vi "setup-camera-acquisition.vi"(9 "Image Size":T3={"H Bin"=1.0, "V Bin"=1.0, "Left"=1.0, "Right"=1024.0, "Top"=1.0, "Bottom"=1024.0} {"V Bin" min=0.0; "H Bin" min=0.0 step=1.0}, 10 "Laser Shutter":T6, 11 "Acquisition Parameters":T5={"Readout Mode"=enum."Image", "Set Acquisition Mode"=enum."Run till abort", "Trigger Mode"=enum."Internal", "Exposure Time (sec)"=0.3, "Accumulation Cycle (s)"=1.0, "Kinetic Cycle Time (s)"=0.0, "Number of Kinetics"=1, "Number of Accumulations"=1, "Set VS Speed"=6.5, "Pixel Rate"=enum."EM CCD 1 Mhz 16 bits", "V Shift Amplitude"=enum."normal", "Preamp Gain"=enum."2.4", "Single Track Settings"={"centre"=0, "height"=1}, "EM CCD Gain"=300, "High Capacity?"=FALSE} {"EM CCD Gain" scale=0.01..300.0; "Single Track Settings"."centre" min=0 max=1024; "Single Track Settings"."height" min=1 max=1024; "Exposure Time (sec)" scale=0.001..10.0 scale format="%#_1g"; "Set VS Speed" min=0.0 format="%#_2f"}) -> (0 "Error Out":errorcluster, 1 "Continue with \nacquisition?":bool, 2 "Image Size Out":T2, 3 "File properties":T4)   [LabVIEW 2014]
uses:
  Shutter Control/Shutter SubVIs/ctts/laser shutters.ctl
  SubVIs/ctt's/Camera Setup Acquisition.ctl
  SubVIs/ctt's/Image size and binning.ctl
  Shutter Control/Shutter SubVIs/ctts/user event shutter global.ctl
  SubVIs/ctt's/image-acquision 2.ctl
  SubVIs/Globals/Initilize Globals.vi
panel:
  out "Pixels Out":i32[](array[numeric])
  in  "Preview Type":T1(radio)
  out "Y Pixel Size":u16
  out "X Pixel Size":u16
  in  "Adjust Image Size":bool
  in  "Set to AOI":bool
  in  "Set to 512 x 300":bool
  in  "Set to Maximum":bool
  in  "Number of preview \nwindows":i32=1 min=0 max=10
  in  "End Program?":bool
  in  "Camera \nShutter":bool
  out "Image":T7(plugin-control)
  # "Exit Parameters"
  # "****Configure Prior to Running Program****"
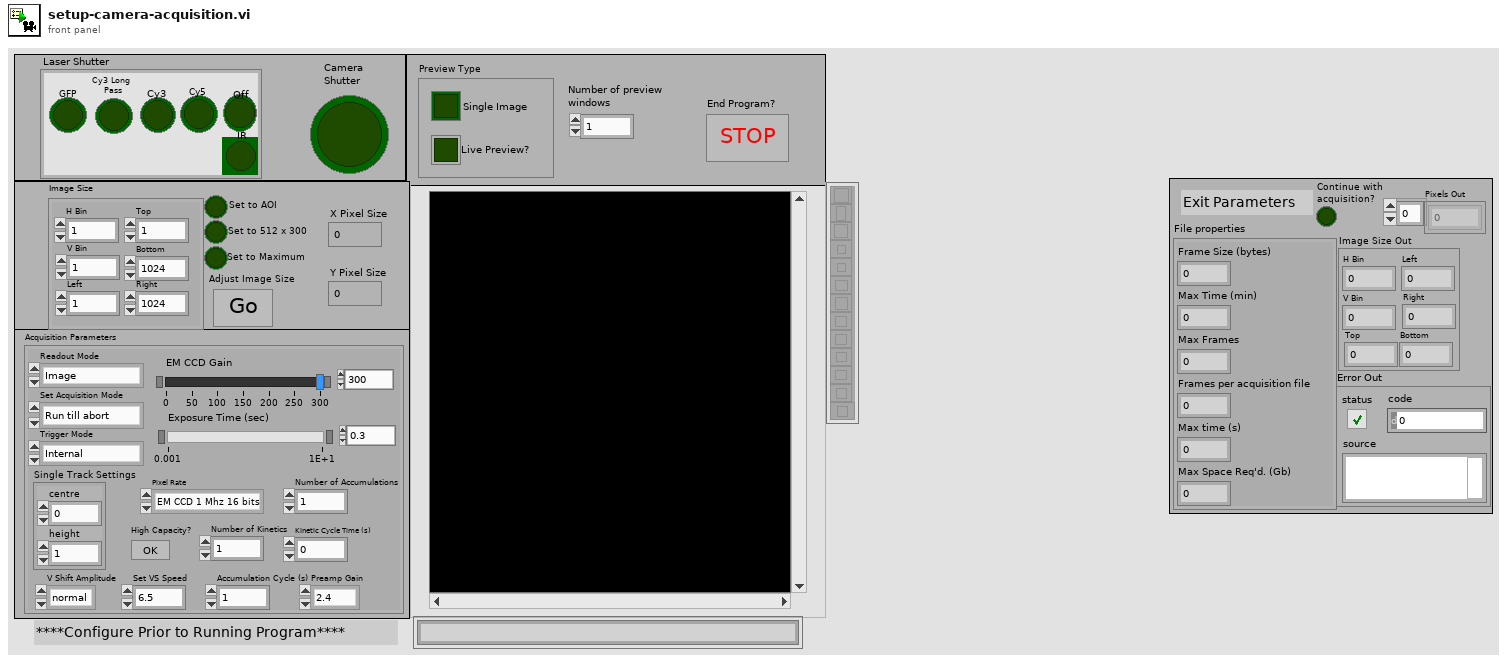
[diagram p1: front panel]
types:
  T1 = enum32{"No Selection", "Live Preview?", "Single Image"}
  T2 = cluster{"H Bin":dbl, "V Bin":dbl, "Left":dbl, "Right":dbl, "Top":dbl, "Bottom":dbl}
  T3 = typedef "Image size and binning.ctl" = cluster{"H Bin":dbl, "V Bin":dbl, "Left":dbl, "Right":dbl, "Top":dbl, "Bottom":dbl}
  T4 = cluster{"Frame Size (bytes)":i32, "Max Time (min)":i32, "Max Frames":i32, "Frames per acquisition file":i32, "Max time (s)":i32, "Max Space Req'd. (Gb)":dbl}
  T5 = typedef "Camera Setup Acquisition.ctl" = cluster{"Readout Mode":enum16{"Full Vertical Binning", "Multi-Track", "Random-Track", "Single-Track", "Image"}, "Set Acquisition Mode":enum16{"(do nothing)", "Single Scan", "Accumulate", "Kinetics", "Fast Kinetics", "Run till abort"}, "Trigger Mode":enum16{"Internal", "External"}, "Exposure Time (sec)":sgl, "Accumulation Cycle (s)":dbl, "Kinetic Cycle Time (s)":dbl, "Number of Kinetics":i32, "Number of Accumulations":i32, "Set VS Speed":dbl, "Pixel Rate":enum16{"EM CCD 10 Mhz 14 bits", "EM CCD 5 Mhz 14 bits", "EM CCD 3 Mhz 14 bits", "EM CCD 1 Mhz 16 bits", "Standard CCD 3 Mhz 14 bits", "Standard CCD 1 Mhz 16 bits"}, "V Shift Amplitude":enum16{"normal", "+1", "+2", "+3", "+4"}, "Preamp Gain":enum16{"1.0", "2.4", "5.0"}, "Single Track Settings":cluster{"centre":i32, "height":i32}, "EM CCD Gain":u16, "High Capacity?":bool}
  T6 = typedef "laser shutters.ctl" = enum32{"No Selection", "GFP", "Cy3 Long \nPass", "Cy3", "Cy5", "Off", "IR"}
  T7 = typedef "IMAQ Image.ctl" = refnum<image>
  T8 = enum32{"Invalid", "Standard", "Closed", "Hidden", "Minimized", "Maximized"}
  T9 = typedef "user event shutter global.ctl" = cluster{"Camera Shutter":bool, "Laser Shutter":enum32{"No Selection", "GFP", "Cy3 Long \nPass", "Cy3", "Cy5", "Off", "IR"}}
  T10 = enum32{"No Selection", "GFP", "Cy3 Long \nPass", "Cy3", "Cy5", "Off", "IR"}
  T11 = typedef "image-acquision 2.ctl" = u32
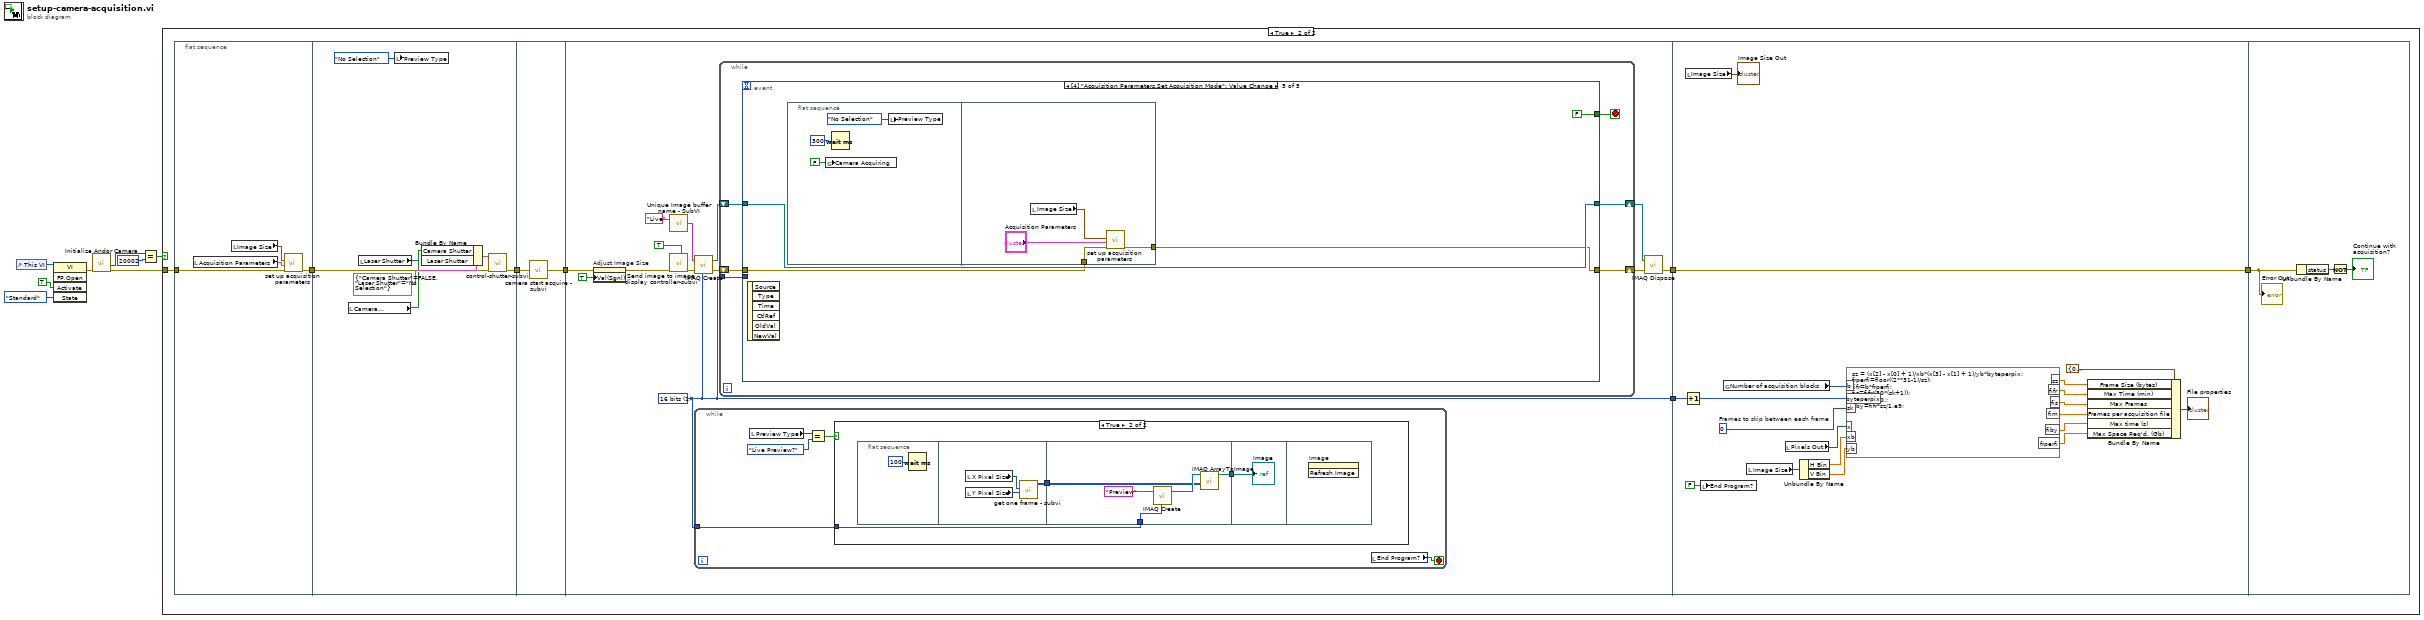
[diagram p0: block diagram]
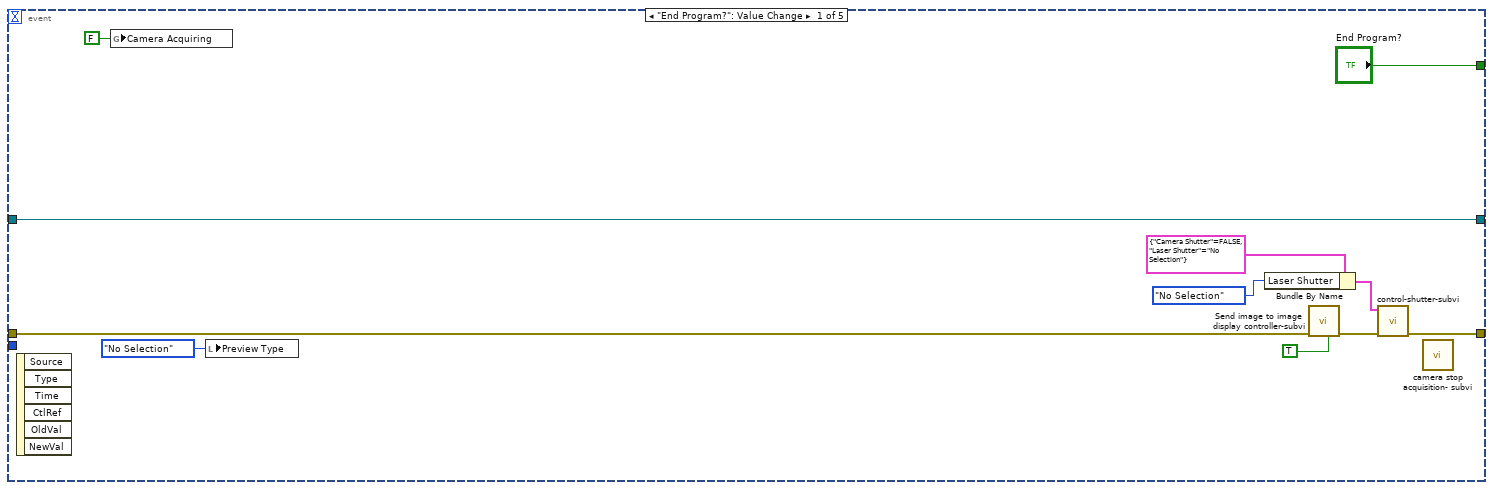
[diagram p4: hidden frame]
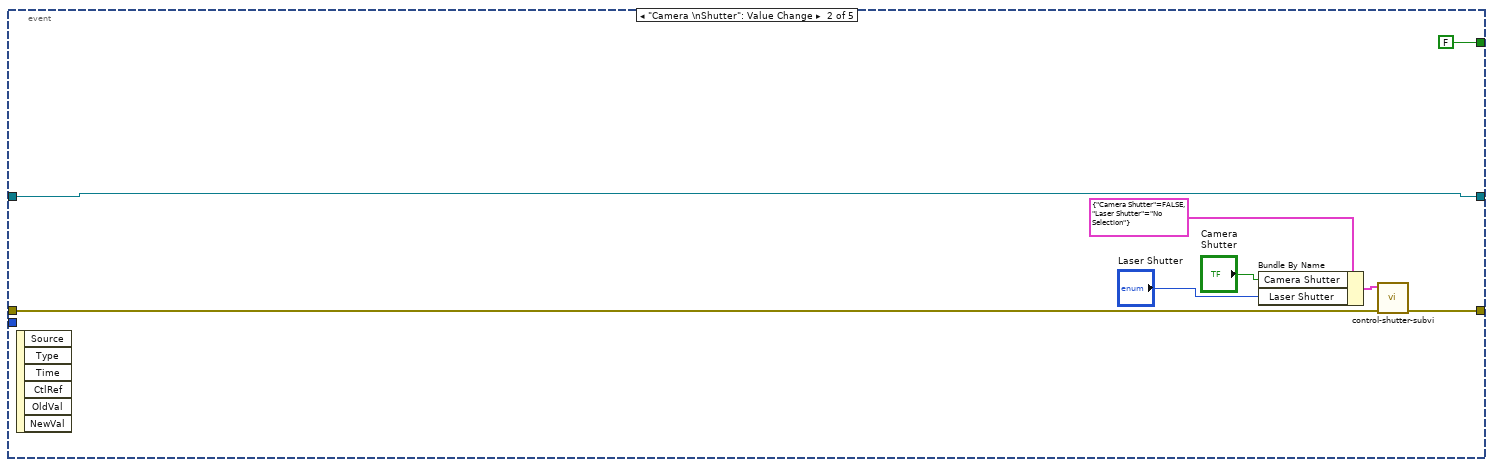
[diagram p5: hidden frame]
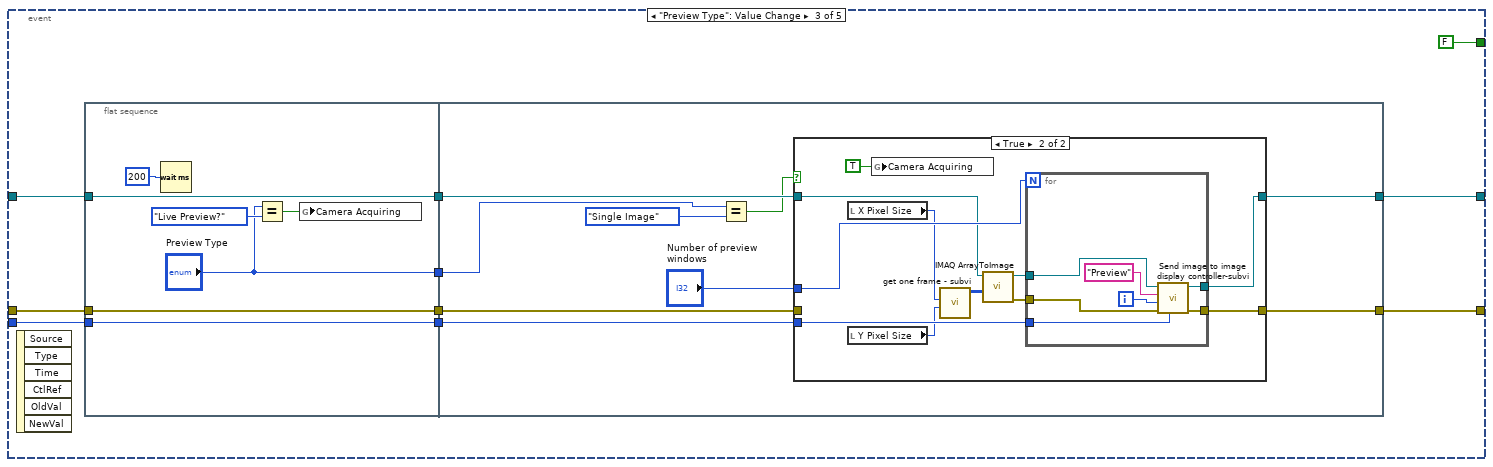
[diagram p6: hidden frame]
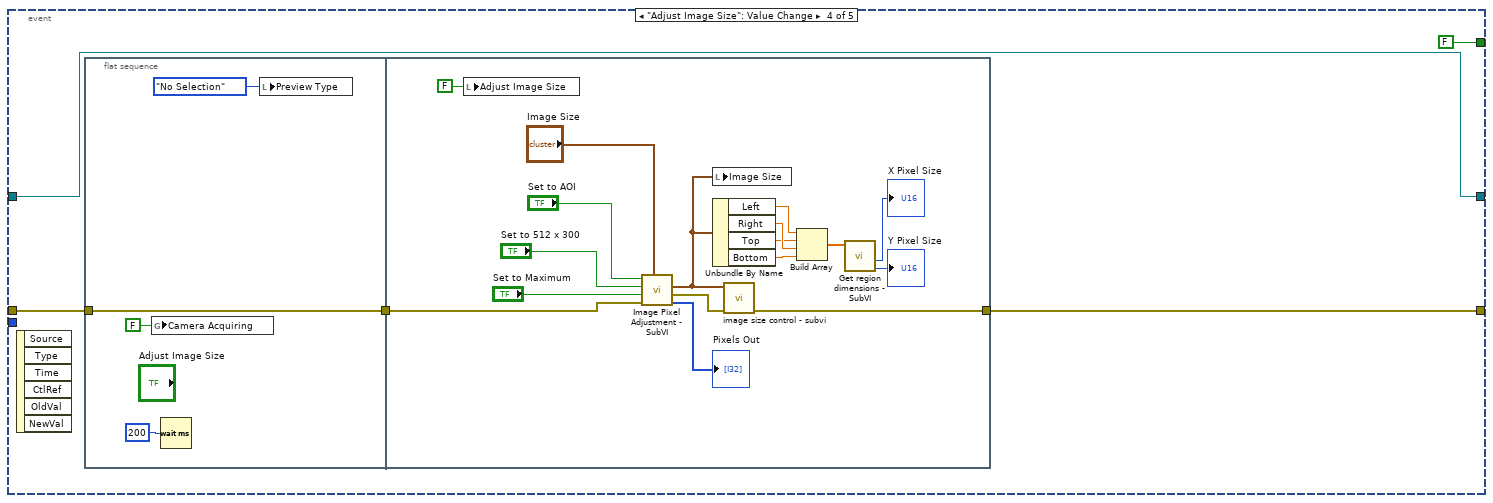
[diagram p8: hidden frame]
diagram:
  n1 = control-ref of="This VI"() -> (w8:refnum<vi>)
  n2 = invoke class="VI" method="FP.Open"(reference=w8, "Activate"=TRUE ("Activate?"), "State"=T8."Standard") -> (error out=w5:errorcluster)  [unwired: 2 in, 4 out]
  n3 = call "Initialize Andor Camera.vi"("error in (no error)"=w5) -> ("Error Out 2"=w1:errorcluster, "Drv Success?"=w4:i32)  [unwired: 9 in]
  n4 = Equal?(x=w4, y=20002) -> (x = y?=w2:bool)
  n5 = case shown="True" w2 {
    tunnel: w1 -> [_ w9]
    frame False {
    }
    frame True {
      n6 = flat-sequence {
        tunnel: [w18] -> w15
        tunnel: w9 -> [w17]
        tunnel: [w22] -> w14
        tunnel: w15 -> [w21]
        tunnel: w14 -> [w28]
        tunnel: [w27] -> w13
        tunnel: [w29] -> w12
        tunnel: w13 -> [w38]
        tunnel: [w40] -> w11
        tunnel: w12 -> [w184]
        tunnel: [w170] -> w10
        tunnel: w11 -> [w170]
        tunnel: w10 -> [w187]
        frame #0 {
          n7 = local read "Acquisition Parameters"() -> (w16:T5)
          n8 = local read "Image Size"() -> (w19:T3)
          n9 = call "set up acquisition parameters.vi"("error in (no error)"=w17, "Acquisition Parameters"=w16, "Image Size"=w19) -> ("error out"=w18:errorcluster)  [unwired: 3 in, 3 out]
        }
        frame #1 {
          n10 = local read "Camera \nShutter"() -> (w24:bool)
          n11 = local read "Laser Shutter"() -> (w23:T6)
          n12 = local write "Preview Type"(T1."No Selection" ("Preview Type")) -> ()
          n13 = Bundle By Name(cluster=T9 {"Camera Shutter"=FALSE, "Laser Shutter"=enum."No Selection"} ("Shutter Control"), "Camera Shutter"=w24, "Laser Shutter"=w23) -> (w25:T9)
          n14 = call "control-shutter-subvi.vi"("Error In"=w21, "Shutter Control"=w25) -> ("Error Out"=w22:errorcluster)  [unwired: 9 in]
        }
        frame #2 {
          n15 = call "camera start acquire - subvi.vi"("error in"=w28) -> ("error out"=w27:errorcluster)
        }
        frame #3 {
          w29 = T11 1 items=["8 bits", "16 bits", "Float", "Complex", "RGB", "HSL"] ("Image Type")
          n16 = property on="Adjust Image Size" class="Bool (strict)"(error in=w38, "Val(Sgnl)"=TRUE ("Value (Signaling)")) -> (error out=w32:errorcluster)  [unwired: 1 in, 1 out]
          n17 = call "Unique Image buffer name - SubVI.vi"("Buffer  base name"="Live") -> ("Image Name"=w35:string)  [unwired: 1 in]
          n18 = call "Send image to image display controller-subvi.vi"("error in"=w32, "Start display controller?"=TRUE) -> ("error out"=w31:errorcluster)  [unwired: 7 in, 1 out]
          n19 = call "IMAQ Create"("Image Name"=w35, "Image Type"=w29, "error in (no error)"=w31) -> ("New Image"=w33:T7, "error out"=w34:errorcluster)  [unwired: 1 in, 1 out]
          n20 = while {
            tunnel: w29 -> [w42]
            stop <- w46 stop-if-true
            n21 = local read "Preview Type"() -> (w45:T1)
            n22 = Equal?(x=w45, y=T1."Live Preview?" ("Preview Type")) -> (x = y?=w44:bool)
            n23 = case shown="True" w44 {
              tunnel: w42 -> [_ w47]
              frame False {
              }
              frame True {
                n24 = flat-sequence {
                  tunnel: [w51] -> w48
                  tunnel: [w56] -> w49
                  tunnel: w48 -> [w55]
                  tunnel: w47 -> [w54]
                  tunnel: w49 -> [w59]
                  frame #0 {
                    n25 = Wait (ms)(milliseconds to wait=u32 100) -> ()  [unwired: 1 out]
                  }
                  frame #1 {
                    n26 = local read "X Pixel Size"() -> (w52:u16)
                    n27 = local read "Y Pixel Size"() -> (w53:u16)
                    n28 = call "get one frame - subvi.vi"("Image Height"=w53, "Image Width"=w52) -> ("Image Array"=w51:i32[][])  [unwired: 9 in]
                  }
                  frame #2 {
                    n29 = call "IMAQ Create"("Image Name"="Preview", "Image Type"=w54) -> ("New Image"=w57:T7)  [unwired: 3 in, 1 out]
                    n30 = call "IMAQ ArrayToImage"("Image Pixels (I16)"=w55, "Image"=w57) -> ("Image Out"=w56:T7)  [unwired: 8 in, 1 out]
                  }
                  frame #3 {
                    "Image" <- w59
                  }
                  frame #4 {
                    n31 = invoke on="Image" class="ImageControl" method="Refresh Image"() -> ()  [unwired: 3 in, 3 out]
                  }
                }
              }
            }
            n32 = local read "End Program?"() -> (w46:bool)
          }
          n33 = while {
            tunnel: w29 -> [w64]
            shift-right: [w61] -> w41
            shift-left: w34 -> [w62]
            shift-right: [w60] -> w37
            shift-left: w33 -> [w63]
            stop <- w65 stop-if-true
            n34 = event shown="[4] \"Acquisition Parameters.Set Acquisition Mode\": Value Change" {
              selector: _ -> [_ _ _ _ _]
              dyn-events: _ -> [_ _ _ _ _]
              timeout: _ -> [_ _ _ _ _]
              tunnel: ["End Program?" FALSE ("Stop Preview?") FALSE ("Stop Preview?") FALSE ("Stop Preview?") FALSE ("Stop Preview?")] -> w65
              tunnel: w64 -> [_ _ w94 _ _]
              tunnel: w63 -> [w75 w77 w93 w134 w160]
              tunnel: [w75 w77 w91 w134 w160] -> w60
              tunnel: w62 -> [w74 w79 w89 w133 w158]
              tunnel: [w66 w78 w90 w132 w157] -> w61
              event "End Program?": Value Change {
                n35 = event-data() -> ()  [unwired: 1 in, 6 out]
                n36 = global write "Initilize Globals.vi" "Camera Acquiring"(FALSE) -> ()
                n37 = local write "Preview Type"(T1."No Selection" ("Preview Type")) -> ()
                n38 = Bundle By Name(cluster=T9 {"Camera Shutter"=FALSE, "Laser Shutter"=enum."No Selection"} ("Shutter Control"), "Laser Shutter"=T10."No Selection") -> (w68:T9)
                n39 = call "Send image to image display controller-subvi.vi"("error in"=w74, "Quit display controller?"=TRUE) -> ("error out"=w67:errorcluster)  [unwired: 7 in, 1 out]
                n40 = call "control-shutter-subvi.vi"("Error In"=w67, "Shutter Control"=w68) -> ("Error Out"=w66:errorcluster)  [unwired: 9 in]
                n41 = call "camera stop acquisition- subvi.vi"() -> ()  [unwired: 1 in]
              }
              event "Camera \nShutter": Value Change {
                n42 = event-data() -> ()  [unwired: 1 in, 6 out]
                n43 = Bundle By Name(cluster=T9 {"Camera Shutter"=FALSE, "Laser Shutter"=enum."No Selection"} ("Shutter Control"), "Camera Shutter"="Camera \nShutter", "Laser Shutter"="Laser Shutter") -> (w81:T9)
                n44 = call "control-shutter-subvi.vi"("Error In"=w79, "Shutter Control"=w81) -> ("Error Out"=w78:errorcluster)  [unwired: 9 in]
              }
              event "Preview Type": Value Change {
                n45 = event-data() -> ()  [unwired: 1 in, 6 out]
                n46 = flat-sequence {
                  tunnel: w89 -> [w99]
                  tunnel: w93 -> [w100]
                  tunnel: w94 -> [w101]
                  tunnel: [w101] -> w88
                  tunnel: [w100] -> w87
                  tunnel: [w99] -> w86
                  tunnel: ["Preview Type"] -> w85
                  tunnel: [w107] -> w91
                  tunnel: [w106] -> w90
                  tunnel: w88 -> [w110]
                  tunnel: w87 -> [w109]
                  tunnel: w86 -> [w105]
                  tunnel: w85 -> [w102]
                  frame #0 {
                    n47 = Wait (ms)(milliseconds to wait=u32 200) -> ()  [unwired: 1 out]
                    n48 = Equal?(x="Preview Type", y=T1."Live Preview?" ("Preview Type")) -> (x = y?=w95:bool)
                    n49 = global write "Initilize Globals.vi" "Camera Acquiring"(w95) -> ()
                  }
                  frame #1 {
                    n50 = Equal?(x=w102, y=T1."Single Image" ("Preview Type")) -> (x = y?=w104:bool)
                    n51 = case shown="True" w104 {
                      tunnel: w110 -> [_ w122]
                      tunnel: w109 -> [w112 w119]
                      tunnel: "Number of preview \nwindows" -> [_ w123]
                      tunnel: [w112 w120] -> w107
                      tunnel: [w111 w121] -> w106
                      tunnel: w105 -> [w111 _]
                      frame False {
                      }
                      frame True {
                        n52 = local read "X Pixel Size"() -> (w115:u16)
                        n53 = local read "Y Pixel Size"() -> (w114:u16)
                        n54 = global write "Initilize Globals.vi" "Camera Acquiring"(TRUE ("Camera Acquiring")) -> ()
                        n55 = call "get one frame - subvi.vi"("Image Height"=w114, "Image Width"=w115) -> ("Image Array"=w116:i32[][])  [unwired: 9 in]
                        n56 = call "IMAQ ArrayToImage"("Image Pixels (I16)"=w116, "Image"=w119) -> ("error out"=w117:errorcluster, "Image Out"=w118:T7)  [unwired: 4 in, 4 out]
                        n57 = for {
                          N: w123 -> [_]
                          tunnel: [w130] -> w121
                          tunnel: w117 -> [w129]
                          tunnel: w118 -> [w128]
                          tunnel: w122 -> [w126]
                          tunnel: [w125] -> w120
                          i -> [w127]
                          n58 = call "Send image to image display controller-subvi.vi"("Image"=w128, "Window Title"="Preview", "Window Number"=w127, "error in"=w129, "Image Type"=w126) -> ("Image Out"=w125:T7, "error out"=w130:errorcluster)  [unwired: 4 in]
                        }
                      }
                    }
                  }
                }
              }
              event "Adjust Image Size": Value Change {
                n59 = event-data() -> ()  [unwired: 1 in, 6 out]
                n60 = flat-sequence {
                  tunnel: w133 -> [w139]
                  tunnel: [w139] -> w131
                  tunnel: [w155] -> w132
                  tunnel: w131 -> [w156]
                  frame #0 {
                    n61 = global write "Initilize Globals.vi" "Camera Acquiring"(FALSE) -> ()
                    n62 = Wait (ms)(milliseconds to wait=u32 200) -> ()  [unwired: 1 out]
                    n63 = local write "Preview Type"(T1."No Selection" ("Preview Type")) -> ()
                  }
                  frame #1 {
                    n64 = local write "Adjust Image Size"(FALSE ("Adjust Image Size")) -> ()
                    n65 = call "Image Pixel Adjustment - SubVI.vi"("Image Size"="Image Size", "error in"=w156, "Set to Maximum"="Set to Maximum", "Set to 512 x 300"="Set to 512 x 300", "Set to AOI"="Set to AOI") -> ("Pixels Out"=→"Pixels Out":i32[], "Error Out (no error)"=w149:errorcluster, "Image Size 2"=w148:T2)  [unwired: 4 in]
                    n66 = local write "Image Size"(w148) -> ()
                    n67 = Unbundle By Name(w148) -> ("Left"=w146:dbl, "Right"=w141:dbl, "Top"=w140:dbl, "Bottom"=w147:dbl)
                    n68 = call "image size control - subvi.vi"("error in (no error)"=w149, "Image Size"=w148) -> ("error out"=w155:errorcluster)  [unwired: 9 in]
                    n69 = Build Array(w146, w140, w141, w147) -> (w145:dbl[])
                    n70 = call "Get region dimensions - SubVI.vi"("x1y1x2y2"=w145) -> ("y size"=→"Y Pixel Size":u16, "x size"=→"X Pixel Size":u16)  [unwired: 7 in, 2 out]
                  }
                }
              }
              event Value Change {
                n71 = event-data() -> ()  [unwired: 1 in, 6 out]
                n72 = flat-sequence {
                  tunnel: w158 -> [w165]
                  tunnel: [w164] -> w157
                  frame #0 {
                    n73 = global write "Initilize Globals.vi" "Camera Acquiring"(FALSE) -> ()
                    n74 = Wait (ms)(milliseconds to wait=u32 300) -> ()  [unwired: 1 out]
                    n75 = local write "Preview Type"(T1."No Selection" ("Preview Type")) -> ()
                  }
                  frame #1 {
                    n76 = local read "Image Size"() -> (w167:T3)
                    n77 = call "set up acquisition parameters.vi"("error in (no error)"=w165, "Acquisition Parameters"="Acquisition Parameters", "Image Size"=w167) -> ("error out"=w164:errorcluster)  [unwired: 3 in, 3 out]
                  }
                }
              }
            }
          }
          n78 = call "IMAQ Dispose"("Image"=w37, "error in (no error)"=w41) -> ("error out"=w40:errorcluster)  [unwired: 1 in, 3 out]
        }
        frame #4 {
          w183 = u16 0  # Frames to skip between each frame
          n79 = Increment(x=w184) -> (x+1=w185:T11)
          n80 = local read "Image Size"() -> (→"Image Size Out":T3)
          n81 = local write "End Program?"(FALSE ("End Program?")) -> ()
          n82 = global read "Initilize Globals.vi" "Number of acquisition blocks"() -> (w186:i8)
          n83 = local read "Image Size"() -> (w174:T3)
          n84 = local read "Pixels Out"() -> (w171:i32[])
          n85 = Unbundle By Name(w174) -> ("H Bin"=w173:dbl, "V Bin"=w172:dbl)
          n86 = formula code="sz = (x[2] - x[0] + 1)/xb*(x[3] - x[1] + 1)/yb*byteperpix;\nfrperfi=floor((2**31-1)/sz);\nfifr=b*frperfi;\nfis=fifr/(30*(sk+1));\nfim=fis/60.;\nfiby=fifr*sz/1.e9;"("x"=w171, "b"=w186, "sk"=w183, "xb"=w173, "yb"=w172, "byteperpix"=w185) -> ("sz"=w180:dbl, "fifr"=w179:dbl, "fis"=w178:dbl, "fim"=w177:dbl, "fiby"=w176:dbl, "frperfi"=w175:dbl)
          n87 = Bundle By Name(cluster=T4 {"Frame Size (bytes)"=0, "Max Time (min)"=0, "Max Frames"=0, "Frames per acquisition file"=0, "Max time (s)"=0, "Max Space Req'd. (Gb)"=0.0} ("File properties"), "Frame Size (bytes)"=w180, "Max Time (min)"=w179, "Max Frames"=w178, "Frames per acquisition file"=w177, "Max time (s)"=w176, "Max Space Req'd. (Gb)"=w175) -> (→"File properties":T4)
        }
        frame #5 {
          n88 = Unbundle By Name(w187) -> ("status"=w189:bool)
          n89 = Not(x=w189) -> (.not. x?=→"Continue with \nacquisition?":bool)
          "Error Out" <- w187
        }
      }
    }
  }
